vi "Read Class Data.vi"(8 "error in (no error)":errorcluster, 11 "PPL Class Test Data in":refnum<class "PPL Class Test Data.lvclass">) -> (0 "error out":errorcluster, 1 "Load Failure":string[](array[string]), 2 "Load Success":string[](array[string]), 3 "PPL Class Test Data out":refnum<class "PPL Class Test Data.lvclass">)   [LabVIEW 2020, in "ProjectBuilder.lvlib" / "PPL Class Test Data.lvclass"]
doc: "Write success and fail string arrays to the private data."
uses:
  PPL Class Test Data.lvclass
  PPL Class Test Data.lvclass/PPL Class Test Data.ctl
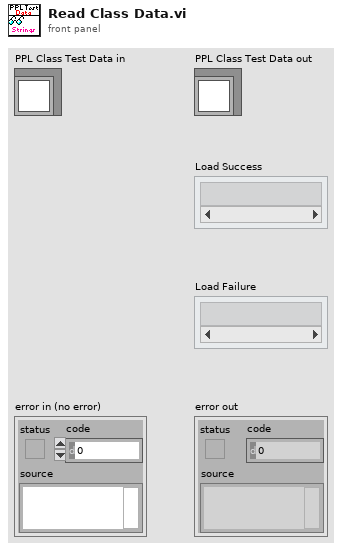
[diagram p1: front panel]
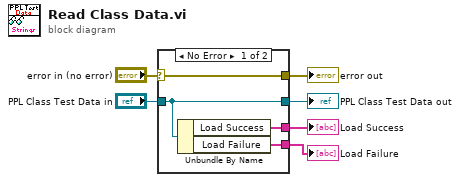
[diagram p0: block diagram]
diagram:
  n1 = case shown="No Error" "error in (no error)" {
    selector: "error in (no error)" -> [w10 w11]
    tunnel: [w10 w11] -> w5
    tunnel: [w9 w12] -> w3
    tunnel: "PPL Class Test Data in" -> [w9 w12]
    tunnel: [w8 _] -> w2
    tunnel: [w7 _] -> w1
    frame No Error {
      n2 = Unbundle By Name(w9) -> ("Load Success"=w8:string[], "Load Failure"=w7:string[])
    }
    frame Error {
    }
  }
  "error out" <- w5
  "PPL Class Test Data out" <- w3
  "Load Success" <- w2
  "Load Failure" <- w1
